vi "MANDAR_BD.vi"(8 "error in (no error)":errorcluster, 9 "BASE DE DATOS":string, 11 "UI_MEX_CAFE_ESPAÑOL in":refnum<class "UI_MEX_CAFE_ESPAÑOL.lvclass">) -> (0 "error out":errorcluster, 3 "UI_MEX_CAFE_ESPAÑOL out":refnum<class "UI_MEX_CAFE_ESPAÑOL.lvclass">)   [LabVIEW 2019, in "UI_MEX_CAFE_ESPAÑOL.lvlib" / "UI_MEX_CAFE_ESPAÑOL.lvclass"]
uses:
  DATABASE_MANEJO/DATABASE_MANEJO Messages/SOLICITAR BASE DE DATOS Msg/SOLICITAR BASE DE DATOS Msg.lvclass/SOLICITAR BASE DE DATOS Msg.ctl
  <vilib>/ActorFramework/Message Enqueuer/Message Enqueuer.lvclass/Message Enqueuer.ctl
  <vilib>/ActorFramework/Message Enqueuer/Enqueue.vi
  DATABASE_MANEJO/DATABASE_MANEJO Messages/SOLICITAR BASE DE DATOS Msg/SOLICITAR BASE DE DATOS Msg.lvclass
  C:/Program Files (x86)/National Instruments/LabVIEW 2019/vi.lib/ActorFramework/Message/Message.lvclass
  <vilib>/ActorFramework/Message Priority Queue/Priority Enqueue.vi
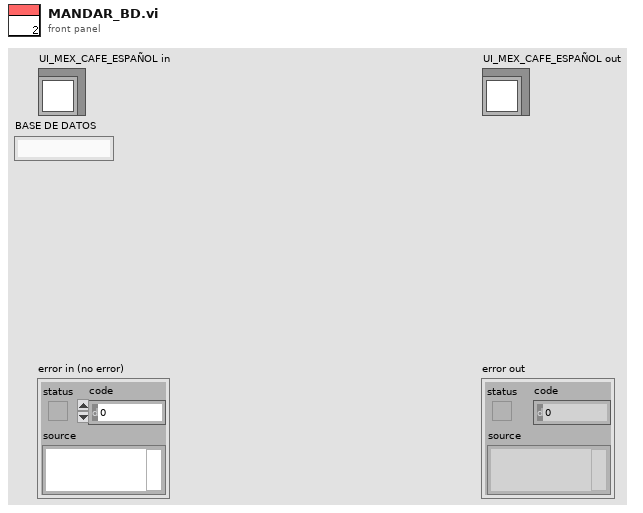
[diagram p1: front panel]
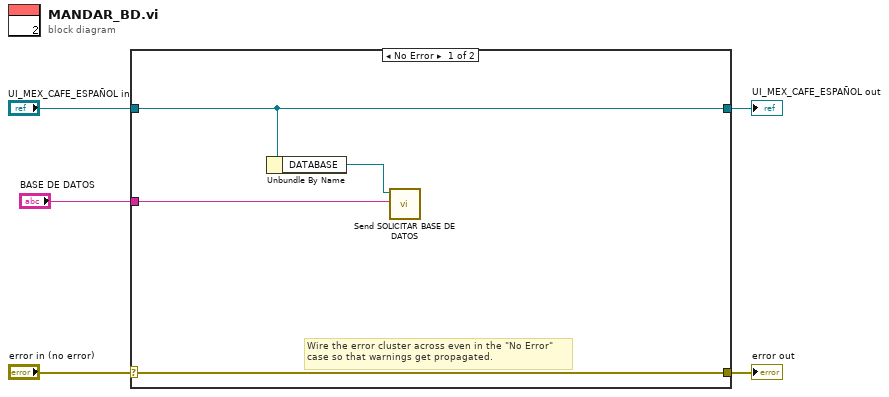
[diagram p0: block diagram]
diagram:
  n1 = case shown="No Error" "error in (no error)" {
    selector: "error in (no error)" -> [w9 w11]
    tunnel: [w9 w11] -> w4
    tunnel: [w8 w10] -> w2
    tunnel: "UI_MEX_CAFE_ESPAÑOL in" -> [w8 w10]
    tunnel: "BASE DE DATOS" -> [w6 _]
    frame No Error {
      # "Wire the error cluster across even in the \"No Error\"\ncase so that warnings get propagated."
      n2 = Unbundle By Name(w8) -> ("DATABASE"=w7:refnum<class "Message Enqueuer.lvclass">)
      n3 = call "Send SOLICITAR BASE DE DATOS.vi"("BASE DE DATOS"=w6, "Message Enqueuer"=w7) -> ()  [unwired: 8 in, 2 out]
    }
    frame Error {
    }
  }
  "error out" <- w4
  "UI_MEX_CAFE_ESPAÑOL out" <- w2
